vi "Test Automatation Example1.vi"() -> ()   [LabVIEW 2025]
uses:
  Typedef/Resource Settings.ctl
  Typedef/TDMS Name Mapping.ctl
panel:
  in  "TDMS File Path":path[](array[path])
  out "Response Passed?":bool[](array[boolean])
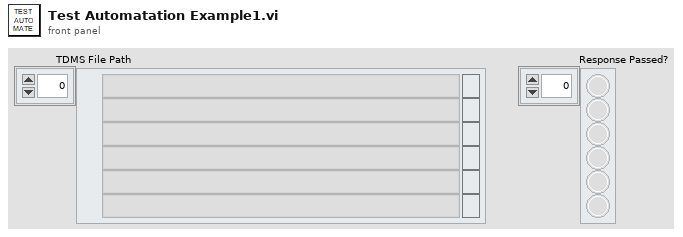
[diagram p1: front panel]
types:
  T1 = cluster{"FGEN Wfm Sequence":string[], "DAQ Wfm Sequence":string[], "Loops":i32[]}
  T2 = typedef "TDMS Name Mapping.ctl" = cluster{"FGEN Channel Mapping":string[][], "DAQ Channel Mapping":string[][], "FGEN Wfm List":string[][], "DAQ Wfm List":string[][]}
  T3 = typedef "Resource Settings.ctl" = cluster{"FGEN Resource":refnum<k15>, "DAQmx Resource":tag, "TDMS File Path":path, "Export Marker0 From File?":bool, "FGEN Gain":dbl, "Scope Resource":refnum<k15>, "Scope Channel":string, "Scope Config File Path":path}
  T4 = cluster{"relativeInitialX":dbl, "xIncrement":dbl, "wfm":dbl[]}[]
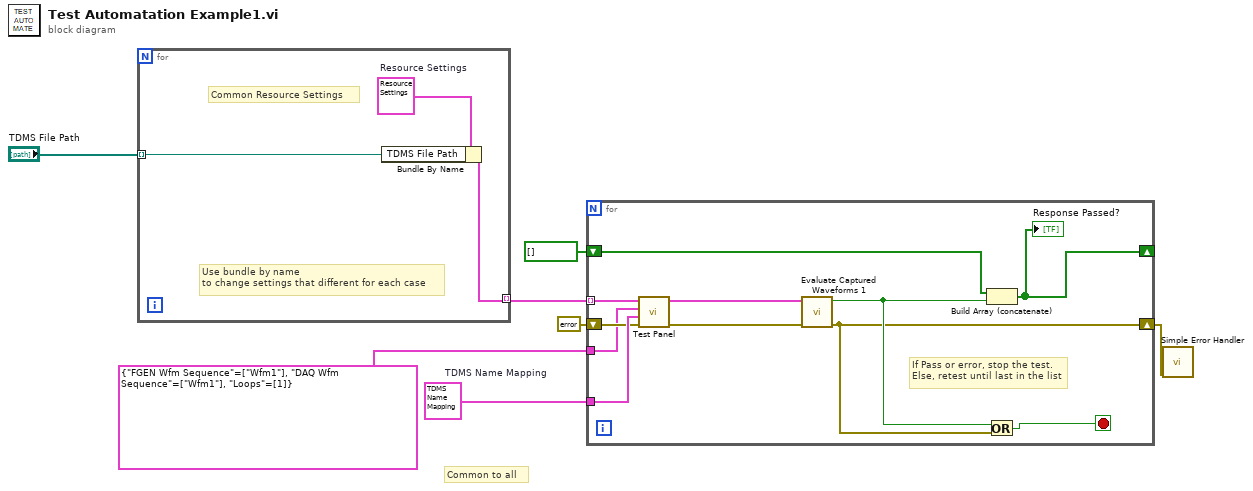
[diagram p0: block diagram]
diagram:
  w7 = T2 {"FGEN Channel Mapping"=[["0", "Chn0"]], "DAQ Channel Mapping"=[["0", "Chn0"], ["1", "Chn1"], ["2", "Chn2"]], "FGEN Wfm List"=[["Wfm1", "FGEN_Wfm1"], ["Wfm2", "FGEN_Wfm2"]], "DAQ Wfm List"=[["Wfm1", "DAQ_Wfm1"], ["Wfm2", "DAQ_Wfm2"]]}  # TDMS Name Mapping
  # "Common to all"
  n1 = for {
    tunnel: [w9] -> w6 mode=indexing
    tunnel: "TDMS File Path" -> [w8] mode=indexing
    w10 = T3 {"FGEN Resource"="", "DAQmx Resource"="", "TDMS File Path"=path "", "Export Marker0 From File?"=TRUE, "FGEN Gain"=1.0, "Scope Resource"="", "Scope Channel"="0", "Scope Config File Path"=path ""}  # Resource Settings
    # "Common Resource Settings"
    # "Use bundle by name\nto change settings that different for each case"
    n2 = Bundle By Name(cluster=w10, "TDMS File Path"=w8) -> (w9:T3)
  }
  n3 = for {
    tunnel: w6 -> [w19] mode=indexing
    tunnel: w7 -> [w18]
    tunnel: T1 {"FGEN Wfm Sequence"=["Wfm1"], "DAQ Wfm Sequence"=["Wfm1"], "Loops"=[1]} ("Wavefom Sequence") -> [w11]
    shift-right: [w15] -> w2
    shift-left: errorcluster {"status"=FALSE, "code"=0, "source"=""} ("error out") -> [w14]
    shift-right: [w12] -> _
    shift-left: bool[] [] -> [w13]
    stop <- w16 stop-if-true
    # "If Pass or error, stop the test.\nElse, retest until last in the list"
    n4 = call "Test Panel.vi"("Error in"=w14, "TDMS Name Mapping"=w18, "Wavefom Sequence"=w11, "Resource Settings"=w19) -> ("Error out"=w20:errorcluster, "Captured Waveforms"=w21:T4)  [unwired: 6 in]
    n5 = call "Evaluate Captured Waveforms 1.vi"("error in"=w20, "Captured Waveforms"=w21) -> ("error out"=w15:errorcluster, "Response Passed?"=w17:bool)  [unwired: 8 in]
    n6 = Build Array (concatenate)(w13, w17) -> (w12:bool[])
    "Response Passed?" <- w12
    n7 = Or(x=w17, y=w15) -> (x .or. y?=w16:bool)
  }
  n8 = call <vilib>:"Simple Error Handler.vi"("error in (no error)"=w2) -> ()  [unwired: 4 in, 5 out]
